vi "Filter Subarray.vi"(10 "Subarray":dbl[](array[numeric]), 11 "Array":dbl[](array[numeric])) -> (3 "Index of Subarray":i32)   [LabVIEW 2017]
doc: "This VI will search and find the <b>Subarray</b> within the <b>Array</b>. It will then return the <b>Index of Subarray</b> where it was found. If the subarray is not found this will be -1.\n\nIt will also return the array as filtered by the subarray if a match is found."
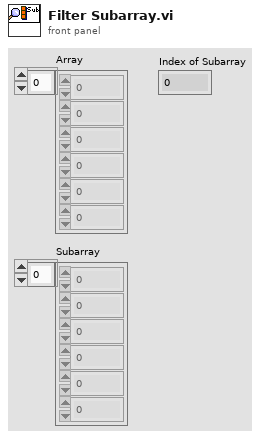
[diagram p1: front panel]
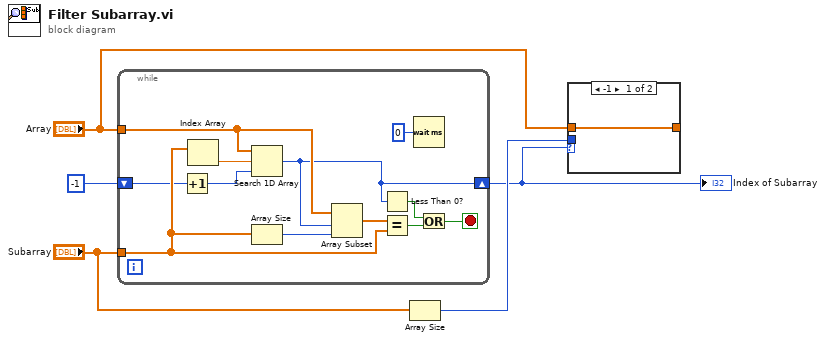
[diagram p0: block diagram]
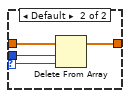
[diagram p2: hidden frame]
diagram:
  n1 = while {
    tunnel: "Array" -> [w16]
    tunnel: "Subarray" -> [w13]
    shift-right: [w9] -> w1
    shift-left: -1 ("index of element") -> [w8]
    stop <- w11 stop-if-true
    n2 = Increment(x=w8) -> (x+1=w7:i32)
    n3 = Index Array(array=w13) -> (element=w17:dbl)  [unwired: 1 in]
    n4 = Search 1D Array(1D array=w16, element=w17, start index (0)=w7) -> (index of element=w9:i32)
    n5 = Array Size(array=w13) -> (size(s)=w15:i32)
    n6 = Array Subset(array=w16, index=w9, length=w15) -> (w14:dbl[])
    n7 = Less Than 0?(x=w9) -> (x < 0?=w12:bool)
    n8 = Equal?(x=w14, y=w13) -> (x = y?=w10:bool)
    n9 = Wait (ms)(milliseconds to wait=u32 0) -> ()  [unwired: 1 out]
    n10 = Or(x=w12, y=w10) -> (x .or. y?=w11:bool)
  }
  "Index of Subarray" <- w1
  n11 = Array Size(array="Subarray") -> (size(s)=w2:i32)
  n12 = case shown="-1" w1 {
    selector: w1 -> [_ w19]
    tunnel: "Array" -> [w18 w22]
    tunnel: w2 -> [_ w21]
    tunnel: [w18 w20] -> _
    frame -1 {
    }
    frame Default {
      n13 = Delete From Array(array=w22, length=w21, index=w19) -> (array with subset deleted=w20:dbl[])  [unwired: 1 out]
    }
  }
